vi "Eval_MultiRes.vi"(8 "error in (no error)":errorcluster, 11 "mupExpr in":refnum<data-value>) -> (0 "error out":errorcluster, 2 "Results":dbl[](array[numeric]) format="%#_13g", 3 "mupExpr out":refnum<data-value>)   [LabVIEW 2015, in "mupExpr.lvclass"]
doc: "Evaluate all expression. Returns one result per expression.\n\nIf the variables are defined for bulk mode evaluation, only the first set (index 0) will be evaluiated."
uses:
  mupExpr.lvclass
  mupExpr.lvclass/mupExpr.ctl
  mupLib/mupCheckError.vi
  mupLib/mupLibPath.vi
  <vilib>/Utility/error.llb/Error Cluster From Error Code.vi
  mupLib/mupLib.lvlib
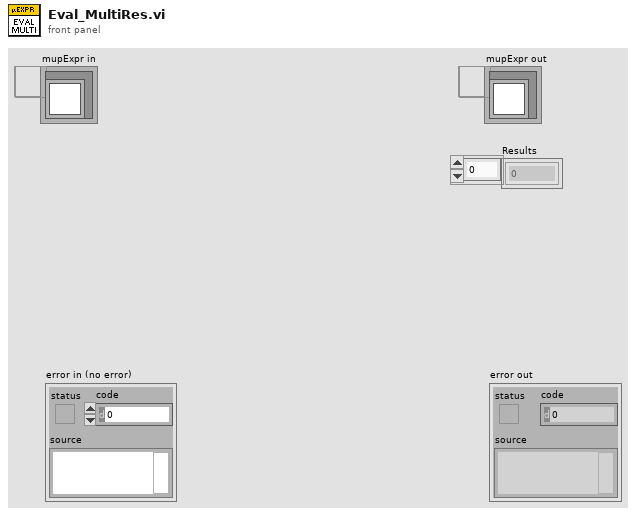
[diagram p1: front panel]
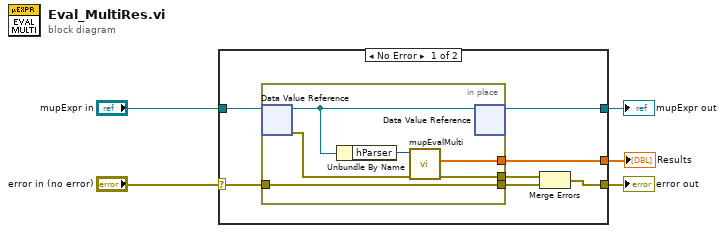
[diagram p0: block diagram]
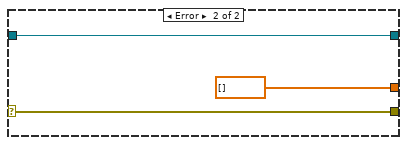
[diagram p2: hidden frame]
diagram:
  n1 = case shown="No Error" "error in (no error)" {
    selector: "error in (no error)" -> [w12 w21]
    tunnel: [w7 w21] -> w4
    tunnel: [w9 w20] -> w2
    tunnel: "mupExpr in" -> [w10 w20]
    tunnel: [w11 dbl[] [] ("return type")] -> w1
    frame No Error {
      n2 = in-place {
        in-place-border: w12 -> [w14]
        in-place-border: [w18] -> w6
        in-place-border: [w13] -> w11
        in-place-border: [w14] -> w8
        n3 = in-place-dvr #1(w10) -> (w16:refnum<class "mupExpr.lvclass">, w15:errorcluster)
        n4 = Unbundle By Name(w16) -> ("hParser"=w17:u64)
        n5 = call "mupEvalMulti.vi"("error in (no error)"=w15, "hParser in"=w17) -> ("error out"=w18:errorcluster, "results"=w13:dbl[])  [unwired: 6 in, 2 out]
        n6 = in-place-dvr #1(w16) -> (w9:refnum<data-value>)  [unwired: 1 out]
      }
      n7 = Merge Errors(w6, w8) -> (w7:errorcluster)
    }
    frame Error {
    }
  }
  "error out" <- w4
  "mupExpr out" <- w2
  "Results" <- w1
